vi "EndOfPathHandler.vi"(6 "CurrentVel":dbl, 8 "MaxAccel":dbl, 9 "MaxVel":dbl, 10 "RobotLocation":cluster{dbl, dbl}, 11 "Path":cluster{"x":dbl, "y":dbl}[](array[cluster])=[{"x"=0.0, "y"=10.0}, {"x"=0.0, "y"=80.0}, {"x"=85.0, "y"=140.0}, {"x"=85.0, "y"=20.0}, {"x"=40.0, "y"=15.0}]) -> (0 "Done":bool, 1 "Override":bool, 2 "ExtraPowerOut":dbl, 3 "VelOut":dbl)   [LabVIEW 2017]
doc: "The end of path handler says when the robot is done traveling the path. It also outputs the velocity the robot should travel at.\n\"But wait!\" you say, \"I thought that was what the MaxVel control was for\". Yes, but the end of path handler outputs 0 vel when the robot gets to the\ndistance it should start deaccelerating (at the END of the PATH). (this vel gets fed into a rate limiter so it obeys max acceleration). This is how it deaccelerates. \n It also outputs a boolean named Override, which tells the robot to stop using a PIDF controller and travel at a constant, slow, speed. This is to try and prevent\nOvershoot at the end. That is a bad solution."
uses:
  <vilib>/addons/control/pid/pid.llb/PID (DBL).vi
  <vilib>/addons/control/pid/NI_PID_pid.lvlib
panel:
  in  "PID gains":T1 {"derivative time (Td, min)" format="%.3f"; "integral time (Ti, min)" format="%.3f"; "proportional gain (Kc)" format="%.3f"}
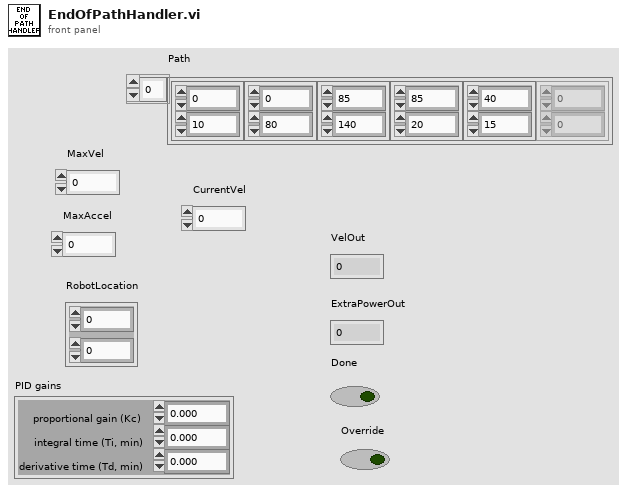
[diagram p1: front panel]
types:
  T1 = cluster{"proportional gain (Kc)":dbl, "integral time (Ti, min)":dbl, "derivative time (Td, min)":dbl}
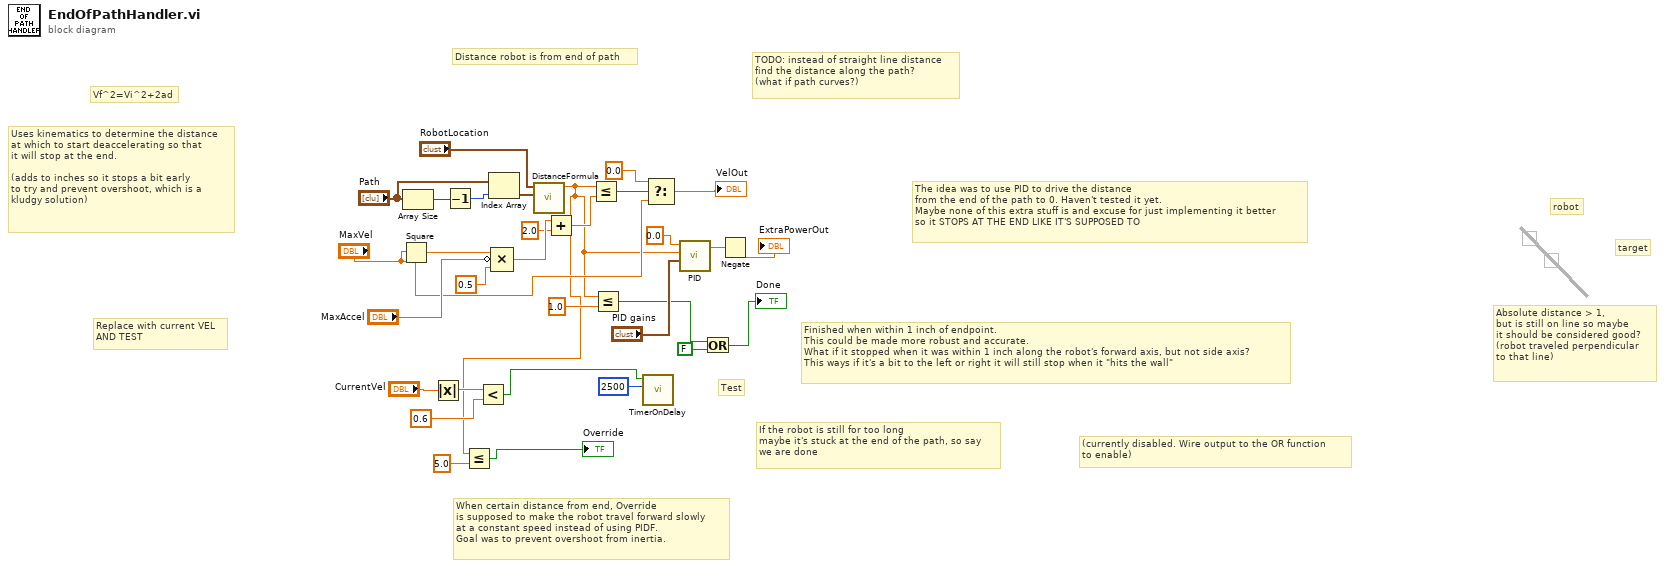
[diagram p0: block diagram]
diagram:
  # "Absolute distance > 1,\nbut is still on line so maybe\nit should be considered good?\n(robot traveled perpendicular\nto that line)"
  # "robot"
  # "target"
  # "Finished when within 1 inch of endpoint.\nThis could be made more robust and accurate.\nWhat if it stopped when it was within 1 inch along the robot's forward axis, but not side axis?\nThis ways if it's a bit to the left or right it will still stop when it \"hits the wall\""
  # "When certain distance from end, Override\nis supposed to make the robot travel forward slowly\nat a constant speed instead of using PIDF.\nGoal was to prevent overshoot from inertia."
  # "(currently disabled. Wire output to the OR function\nto enable)"
  # "If the robot is still for too long\nmaybe it's stuck at the end of the path, so say\nwe are done"
  # "The idea was to use PID to drive the distance\nfrom the end of the path to 0. Haven't tested it yet.\nMaybe none of this extra stuff is and excuse for just implementing it better\nso it STOPS AT THE END LIKE IT'S SUPPOSED TO"
  # "TODO: instead of straight line distance\nfind the distance along the path?\n(what if path curves?)"
  # "Uses kinematics to determine the distance\nat which to start deaccelerating so that\nit will stop at the end.\n\n(adds to inches so it stops a bit early\nto try and prevent overshoot, which is a\nkludgy solution)"
  # "Distance robot is from end of path"
  # "Test"
  # "Replace with current VEL\nAND TEST"
  # "Vf^2=Vi^2+2ad"
  n1 = Square(x="MaxVel") -> (x^2=w31:dbl)
  n2 = Array Size(array="Path") -> (size(s)=w28:i32)
  n3 = Absolute Value(x="CurrentVel") -> (abs(x)=w7:dbl)
  n4 = Decrement(x=w28) -> (x-1=w27:i32)
  n5 = Less?(x=w7, y=0.6) -> (x < y?=w4:bool)
  n6 = Index Array(array="Path", index=w27) -> (element=w25:cluster{"x":dbl, "y":dbl})
  n7 = Compound Arithmetic op=MULTIPLY(w31, invert "MaxAccel", 0.5 ("value")) -> (w13:dbl)
  n8 = call "DistanceFormula.vi"("Point 2"=w25, "Point 1"="RobotLocation") -> ("Distance"=w5:dbl)  [unwired: 9 in]
  n9 = Less Or Equal?(x=w5, y=5.0) -> (x <= y?=→"Override":bool)
  n10 = Add(x=w13, y=2.0) -> (x+y=w11:dbl)
  n11 = Less Or Equal?(x=w5, y=w11) -> (x <= y?=w22:bool)
  n12 = Less Or Equal?(x=w5, y=1.0) -> (x <= y?=w10:bool)
  n13 = call "TimerOnDelay.vi"("Time Limit"=u32 2500, "Input"=w4) -> ()  [unwired: 9 in, 1 out]
  n14 = Select(t=0.0, s=w22, f="MaxVel") -> (s? t:f=→"VelOut":dbl)
  n15 = call-poly <vilib>:"PID.vi"("PID gains"="PID gains", "process variable"=w5, "setpoint"=0.0) -> ("output"=w16:dbl)  [unwired: 7 in, 1 out]
  n16 = Or(x=w10, y=FALSE) -> (x .or. y?=→"Done":bool)
  n17 = Negate(x=w16) -> (-x=→"ExtraPowerOut":dbl)
